vi "Solve2.vi"(8 "Error In":errorcluster, 11 "object in":refnum<class "2022_6.lvclass">) -> (0 "Error Out":errorcluster, 2 "Result":u64, 3 "object out":refnum<class "2022_6.lvclass">)   [LabVIEW 2020, in "2022_6.lvclass"]
uses:
  2022_6.lvclass
  2022_6.lvclass/2022_6.ctl
  528768ee-3f3b-48e1-8191-465e3a11b862.vi
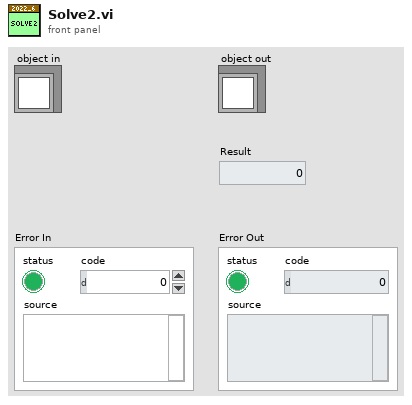
[diagram p1: front panel]
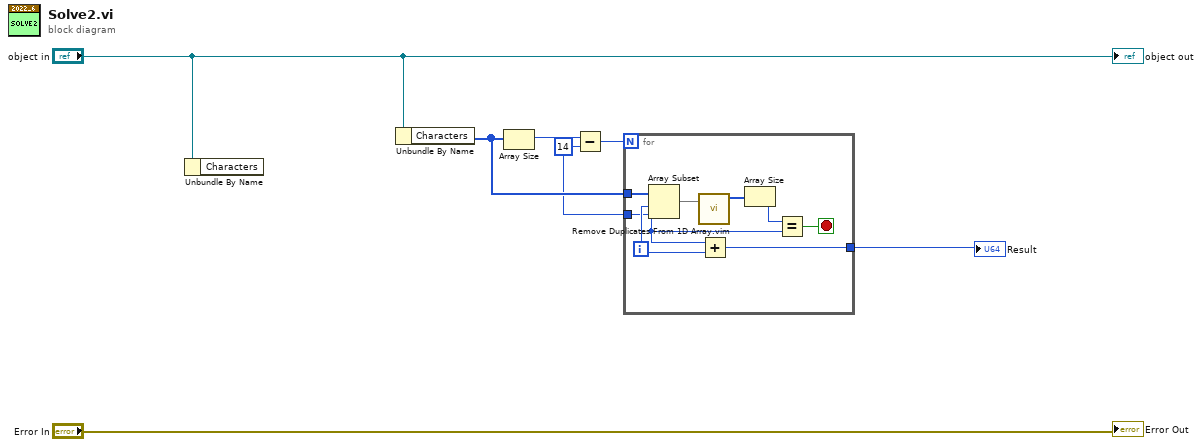
[diagram p0: block diagram]
diagram:
  w3 = 14 ("y")
  n1 = Unbundle By Name("object in") -> ()  [unwired: 1 out]
  n2 = Unbundle By Name("object in") -> ("Characters"=w4:u8[])
  n3 = Array Size(array=w4) -> (size(s)=w6:i32)
  n4 = Subtract(x=w6, y=w3) -> (x-y=w5:i32)
  n5 = for {
    N: w5 -> [_]
    tunnel: w4 -> [w15]
    tunnel: w3 -> [w9]
    tunnel: [w8] -> w1
    i -> [w10]
    stop <- w11 stop-if-true
    n6 = Array Subset(array=w15, index=w10, length=w9) -> (w14:u8[])
    n7 = call "Remove Duplicates From 1D Array.vim"("array"=w14) -> ("array with duplicates removed"=w13:u8[])  [unwired: 10 in]
    n8 = Add(x=w9, y=w10) -> (x+y=w8:i32)
    n9 = Array Size(array=w13) -> (size(s)=w12:i32)
    n10 = Equal?(x=w12, y=w9) -> (x = y?=w11:bool)
  }
  "Result" <- w1
  "Error Out" <- "Error In"
  "object out" <- "object in"
